vi "close.vi"(8 "error in (no error)":errorcluster caption="entrée d'erreur (pas d'erreur)", 11 "hHandle":i32) -> (0 "error out":errorcluster caption="sortie d'erreur")   [LabVIEW 2020, in "usb_relay_device.lvlib"]
doc: "void EXPORT_API usb_relay_device_close(int hHandle);"
uses:
  usb_relay_device.lvlib
  usb_relay_device.dll
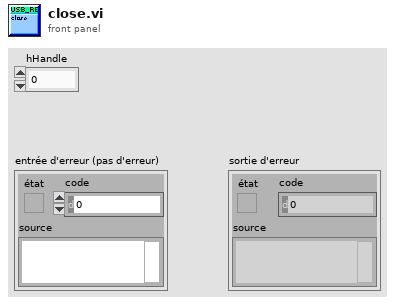
[diagram p1: front panel]
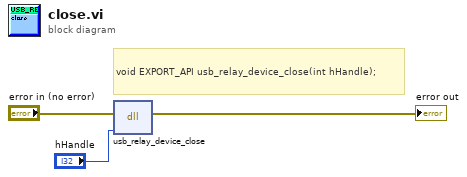
[diagram p0: block diagram]
diagram:
  # "void EXPORT_API usb_relay_device_close(int hHandle);"
  n1 = dll-call lib="C:/Users/ngarcin/OneDrive - Altyor/Standard TB/Class/Relay_Board/Relay_Board usb_Relay_device/usb_relay_device/usb_relay_device.dll" fn="usb_relay_device_close"(error in="error in (no error)", "hHandle"="hHandle") -> (error out=→"error out":errorcluster)  [unwired: 4 in, 1 out]
